vi "test_Create Global MetaData Channel_single channel type cast.vi"(8 "error in (no error)":errorcluster, 11 "TestCase in":refnum<class "Instrument Addon Scripting API Channels Unit Tests.lvclass">) -> (0 "error out":errorcluster, 3 "TestCase out":refnum<class "Instrument Addon Scripting API Channels Unit Tests.lvclass">)   [LabVIEW 2019, in "Instrument Addon Scripting API Channels Unit Tests.lvclass"]
uses:
  Instrument Addon Scripting API Channels Unit Tests.lvclass
  Addon/Addon Shared/Types/FG Control.ctl
  APIs/Scripting API/TypeDefs/Single Channel Type Cast Settings.ctl
  Addon/Addon Shared/Types/Type Cast Type.ctl
  Addon/Addon Shared/Types/Endian.ctl
  Instrument Addon Scripting API Channels Unit Tests.lvclass/Instrument Addon Scripting API Channels Unit Tests.ctl
  Addon/Addon Shared/SubVIs/Constants.vi
  APIs/Scripting API/Channels/Create Global MetaData Channel - Single Channel - Type Cast.vi
  <vilib>/NI VeriStand/Custom Device Tools/Custom Device Utility Library/NI VeriStand - Search for Item by GUID.vi
  <vilib>/NI VeriStand/Custom Device Tools/Custom Device Utility Library/NI VeriStand - Search for Item by Name.vi
  <vilib>/NI VeriStand/Custom Device API/NI VeriStand - Get Item Property.vi
  <vilib>/NI VeriStand/Custom Device API/Get Item Property (U32).vi
  <vilib>/NI VeriStand/Custom Device API/Get Item Property (String Array).vi
  <vilib>/NI VeriStand/Custom Device API/Get Item Property (String).vi
  <vilib>/NI VeriStand/Custom Device API/NI VeriStand - Set Item Property.vi
  <vilib>/NI VeriStand/Custom Device API/Set Item Property (U32).vi
  <vilib>/NI VeriStand/Custom Device API/Set Item Property (String Array).vi
  <vilib>/NI VeriStand/Custom Device API/NI VeriStand - Get Item Children.vi
  Addon/Addon Shared/SubVIs/Set Channel Value Table.vi
  <vilib>/NI VeriStand/Custom Device API/Set Item Property (String).vi
  <vilib>/addons/_JKI Toolkits/VI Tester/TestCase.llb/TestCase.lvclass
  Instrument Addon Scripting API Test Assets/Instrument Addon Scripting API Test Assets.lvclass
  <vilib>/NI VeriStand/Custom Device Tools/Custom Device Utility Library/Custom Device Utility Library.lvlib
  Addon/Addon Shared/Instrument Addon Shared.lvlib
  <vilib>/NI VeriStand/Custom Device API/Custom Device API.lvlib
  APIs/Scripting API/Instrument Addon Scripting API.lvlib
  C:/Program Files (x86)/National Instruments/LabVIEW 2019/vi.lib/addons/_JKI Toolkits/VI Tester/TestCase.llb/TestCase.lvclass
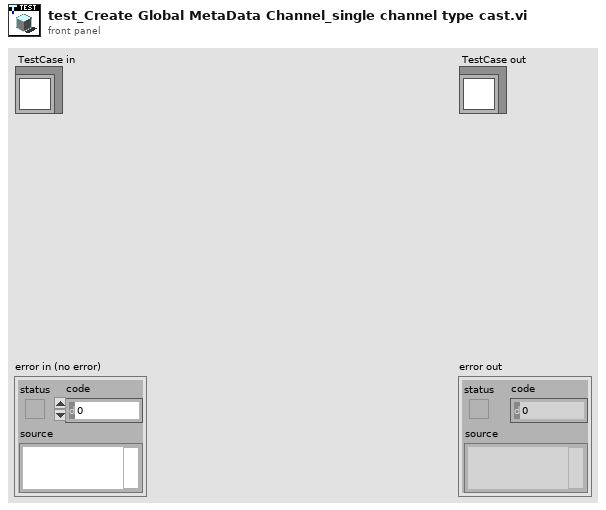
[diagram p1: front panel]
types:
  T1 = typedef "Instrument Addon Shared.lvlib/FG Control.ctl" = enum16{"Get", "Set"}
  T2 = typedef "Instrument Addon Scripting API.lvlib/Single Channel Type Cast Settings.ctl" = cluster{"Default Value":dbl, "Units":string, "Type":T3, "Endian":T4}
  T3 = typedef "Instrument Addon Shared.lvlib/Type Cast Type.ctl" = enum16{"DBL", "SGL", "U64", "U32", "U16", "U8", "I64", "I32", "I16", "I8"}
  T4 = typedef "Instrument Addon Shared.lvlib/Endian.ctl" = enum16{"Native", "Little", "Big"}
  T5 = typedef "Custom Device API.lvlib/Custom Device Item Ref.ctl" = u64
  T6 = typedef "Instrument Addon Shared.lvlib/MetaData Parameters.ctl" = cluster{"Data Type":T7, "Channel Type":T8, "List":string[], "Format String":string, "Type":T3, "Delimiter":string, "Endian":T4}
  T7 = typedef "Instrument Addon Shared.lvlib/Protocol Data Type.ctl" = enum16{"Single Channel", "Array"}
  T8 = typedef "Instrument Addon Shared.lvlib/Metadata Channel Type.ctl" = enum16{"Enumerated List", "Format", "Type Cast"}
  T9 = typedef "Custom Device API.lvlib/Custom Device Channel.ctl" = cluster{"Type":T10, "Units":string, "Default Value":dbl, "Faultable":bool, "Scalable":bool}
  T10 = typedef "Custom Device API.lvlib/Custom Device Channel Type.ctl" = enum16{"Input", "Output"}
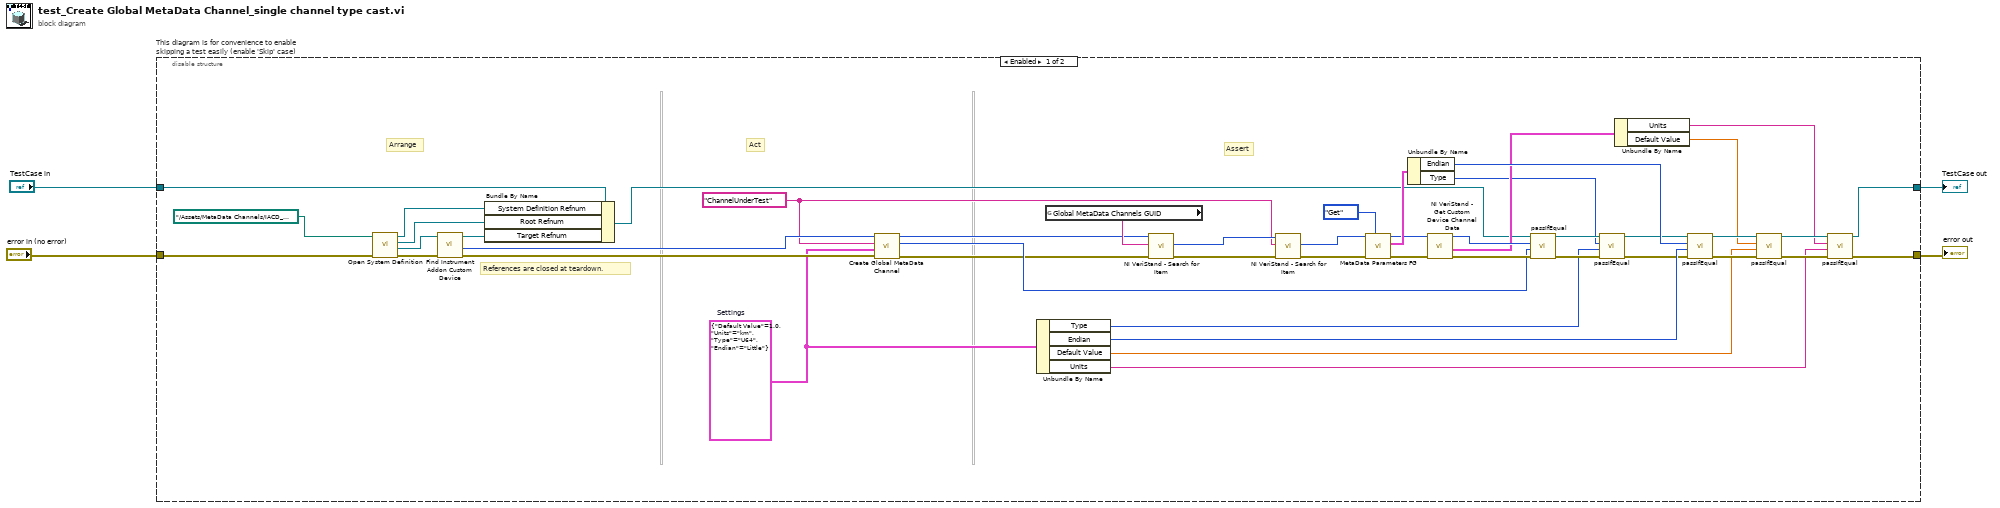
[diagram p0: block diagram]
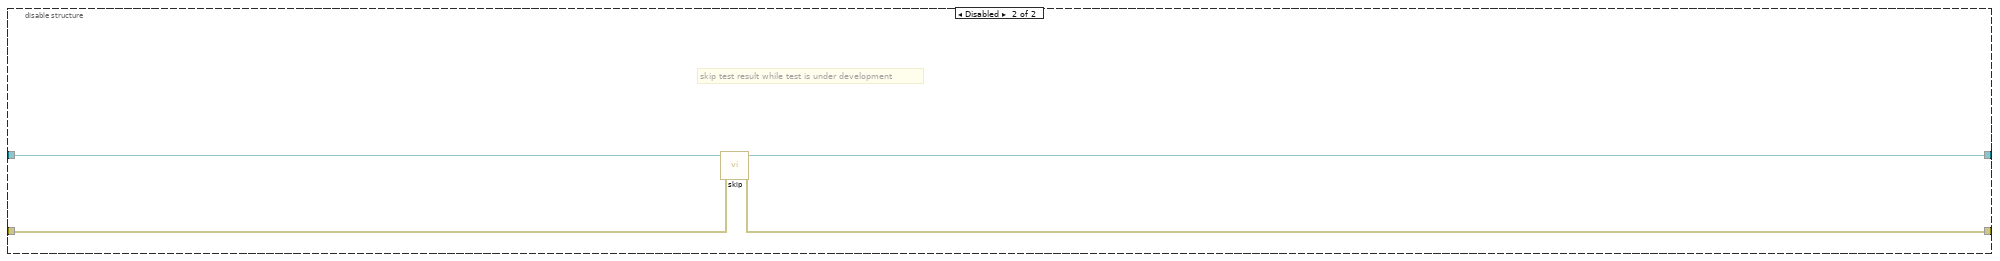
[diagram p2: hidden frame]
diagram:
  n1 = disable-structure "This diagram is for convenience to enable skipping a test easily (enable 'Skip' case)" shown="Enabled" {
    disable-tunnel: "TestCase in" -> [w19 w54]
    disable-tunnel: [w26 w52] -> w1
    disable-tunnel: [w25 w53] -> w3
    disable-tunnel: "error in (no error)" -> [w50 w51]
    frame Enabled {
      w12 = T2 {"Default Value"=1.0, "Units"="km", "Type"=enum."U64", "Endian"=enum."Little"}  # Settings
      w17 = "ChannelUnderTest" ("Name")
      # "References are closed at teardown."
      # "Assert"
      # "Act"
      # "Arrange"
      n2 = call "Open System Definition.vi"("error in (no error)"=w50, "System Definition File"=path "../Assets/MetaData Channels/IACD_channels.nivssdf") -> ("error out"=w48:errorcluster, "Target Refnum"=w49:refnum<k24>, "Root Refnum"=w22:refnum<k24>, "System Definition Refnum"=w21:refnum<k24>)  [unwired: 6 in]
      n3 = call "Find Instrument Addon Custom Device.vi"("error in"=w48, "target in"=w49) -> ("error out"=w16:errorcluster, "NodeID"=w18:u64, "target out"=w23:refnum<k24>)  [unwired: 7 in]
      n4 = Bundle By Name(cluster=w19, "System Definition Refnum"=w21, "Root Refnum"=w22, "Target Refnum"=w23) -> (w20:refnum<class "Instrument Addon Scripting API Channels Unit Tests.lvclass">)
      n5 = call-poly "Create Global MetaData Channel.vi"("error in (no error)"=w16, "settings"=w12, "channel name"=w17, "instrument addon refnum in"=w18) -> ("error out"=w13:errorcluster, "channel refnum"=w14:T5, "instrument addon refnum out"=w15:T5)  [unwired: 5 in]
      n6 = Unbundle By Name(w12) -> ("Type"=w7:T3, "Endian"=w35:T4, "Default Value"=w31:dbl, "Units"=w30:string)
      n7 = global read "Constants.vi" "Global MetaData Channels GUID"() -> (w47:string)
      n8 = call-poly <vilib>:"NI VeriStand - Search for Item.vi"("error in"=w13, "Item GUID"=w47, "Section Ref in"=w15) -> ("error out"=w45:errorcluster, "Item Ref"=w46:T5)  [unwired: 5 in, 2 out]
      n9 = call-poly <vilib>:"NI VeriStand - Search for Item.vi"("error in"=w45, "Item Name"=w17, "Section Ref in"=w46) -> ("error out"=w44:errorcluster, "Item Ref"=w43:T5)  [unwired: 5 in, 2 out]
      n10 = call "MetaData Parameters FG.vi"("Action"=FG_Control."Get", "error in (no error)"=w44, "Item Ref in"=w43) -> ("error out"=w33:errorcluster, "MetaData Parameters"=w41:T6, "Item Ref out"=w34:T5)  [unwired: 6 in]
      n11 = Unbundle By Name(w41) -> ("Endian"=w36:T4, "Type"=w6:T3)
      n12 = call <vilib>:"NI VeriStand - Get Custom Device Channel Data.vi"("error in (no error)"=w33, "Channel Ref in"=w34) -> ("error out"=w24:errorcluster, "Channel"=w29:T9, "Channel Ref out"=w32:T5)  [unwired: 4 in, 3 out]
      n13 = call-dynamic "passIfEqual.vi"("error in (no error)"=w24, "y"=w14, "x"=w32, "TestCase in"=w20) -> ("error out"=w11:errorcluster, "TestCase out"=w9:refnum<class "Instrument Addon Scripting API Channels Unit Tests.lvclass">)  [unwired: 6 in]
      n14 = call-dynamic "passIfEqual.vi"("error in (no error)"=w11, "y"=w7, "x"=w6, "TestCase in"=w9) -> ("error out"=w10:errorcluster, "TestCase out"=w8:refnum<class "Instrument Addon Scripting API Channels Unit Tests.lvclass">)  [unwired: 6 in]
      n15 = Unbundle By Name(w29) -> ("Units"=w27:string, "Default Value"=w28:dbl)
      n16 = call-dynamic "passIfEqual.vi"("error in (no error)"=w10, "y"=w35, "x"=w36, "TestCase in"=w8) -> ("error out"=w40:errorcluster, "TestCase out"=w39:refnum<class "Instrument Addon Scripting API Channels Unit Tests.lvclass">)  [unwired: 6 in]
      n17 = call-dynamic "passIfEqual.vi"("error in (no error)"=w40, "y"=w31, "x"=w28, "TestCase in"=w39) -> ("error out"=w38:errorcluster, "TestCase out"=w37:refnum<class "Instrument Addon Scripting API Channels Unit Tests.lvclass">)  [unwired: 6 in]
      n18 = call-dynamic "passIfEqual.vi"("error in (no error)"=w38, "y"=w30, "x"=w27, "TestCase in"=w37) -> ("error out"=w25:errorcluster, "TestCase out"=w26:refnum<class "Instrument Addon Scripting API Channels Unit Tests.lvclass">)  [unwired: 6 in]
    }
    frame Disabled {
      # "skip test result while test is under development"
      n19 = call <vilib>:"skip.vi"("error in (no error)"=w51, "TestCase in"=w54) -> ("error out"=w53:errorcluster, "TestCase out"=w52:refnum<class "Instrument Addon Scripting API Channels Unit Tests.lvclass">)  [unwired: 8 in]
    }
  }
  "error out" <- w3
  "TestCase out" <- w1
